vi "FlatToRichrouteguide_Rectangle.vi"(5 "OutputClusterType":T1, 11 "InputCluster":T3) -> (3 "OutputCluster":T1)   [LabVIEW 2019, in "route_guide_client.lvlib"]
uses:
  route_guide_client.lvlib
  routeguide_Rectangle_Flat.ctl
  routeguide_Point_Flat.ctl
  routeguide_Rectangle.ctl
  routeguide_Point.ctl
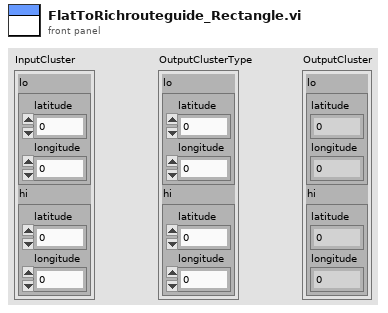
[diagram p1: front panel]
types:
  T1 = typedef "route_guide_client.lvlib/routeguide_Rectangle.ctl" = cluster{"lo":T2, "hi":T2}
  T2 = typedef "route_guide_client.lvlib/routeguide_Point.ctl" = cluster{"latitude":i32, "longitude":i32}
  T3 = typedef "route_guide_client.lvlib/routeguide_Rectangle_Flat.ctl" = cluster{"lo":T4, "hi":T4}
  T4 = typedef "route_guide_client.lvlib/routeguide_Point_Flat.ctl" = cluster{"latitude":i32, "longitude":i32}
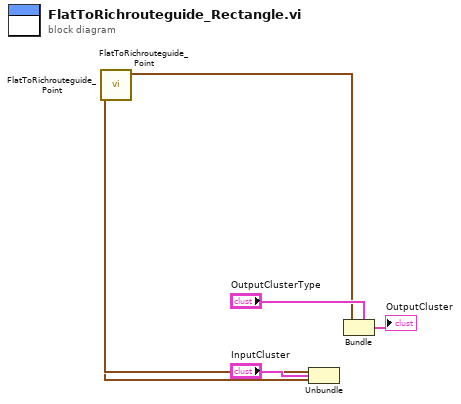
[diagram p0: block diagram]
diagram:
  n1 = Unbundle "Unbundle"("InputCluster") -> ("lo"=w4:T4, "hi"=w2:T4)
  n2 = call "FlatToRichrouteguide_Point.vi"("InputCluster"=w2) -> ("OutputCluster"=w1:T2)  [unwired: 10 in]
  n3 = call "FlatToRichrouteguide_Point.vi"("InputCluster"=w4) -> ("OutputCluster"=w3:T2)  [unwired: 10 in]
  n4 = Bundle "Bundle"(cluster="OutputClusterType", "lo"=w3, "hi"=w1) -> (→"OutputCluster":T1)
